vi "read_signal.vi"(8 "error in (no error)":errorcluster, 9 "Location":i32, 10 "Experiment Settings ID":i32, 11 "Dust Event ID":i32) -> (0 "error out":errorcluster, 3 "Signal Array":T1[](array[typedef]))   [LabVIEW 2012]
uses:
  Public API/Post_Signal.ctl
  Role ID.ctl
  Hardware ID.ctl
  <vilib>/addons/h5labview/H5F_mode.ctl
  <vilib>/addons/h5labview/polymorph/H5A_read_var.vi
  <vilib>/addons/h5labview/H5File.lvlib
  <vilib>/addons/h5labview/H5GroupObject.lvlib
  <vilib>/addons/h5labview/H5Attrib.lvlib
panel:
  out "size(s)":i32
  out "names":string[](array[string])
  # "Signal"
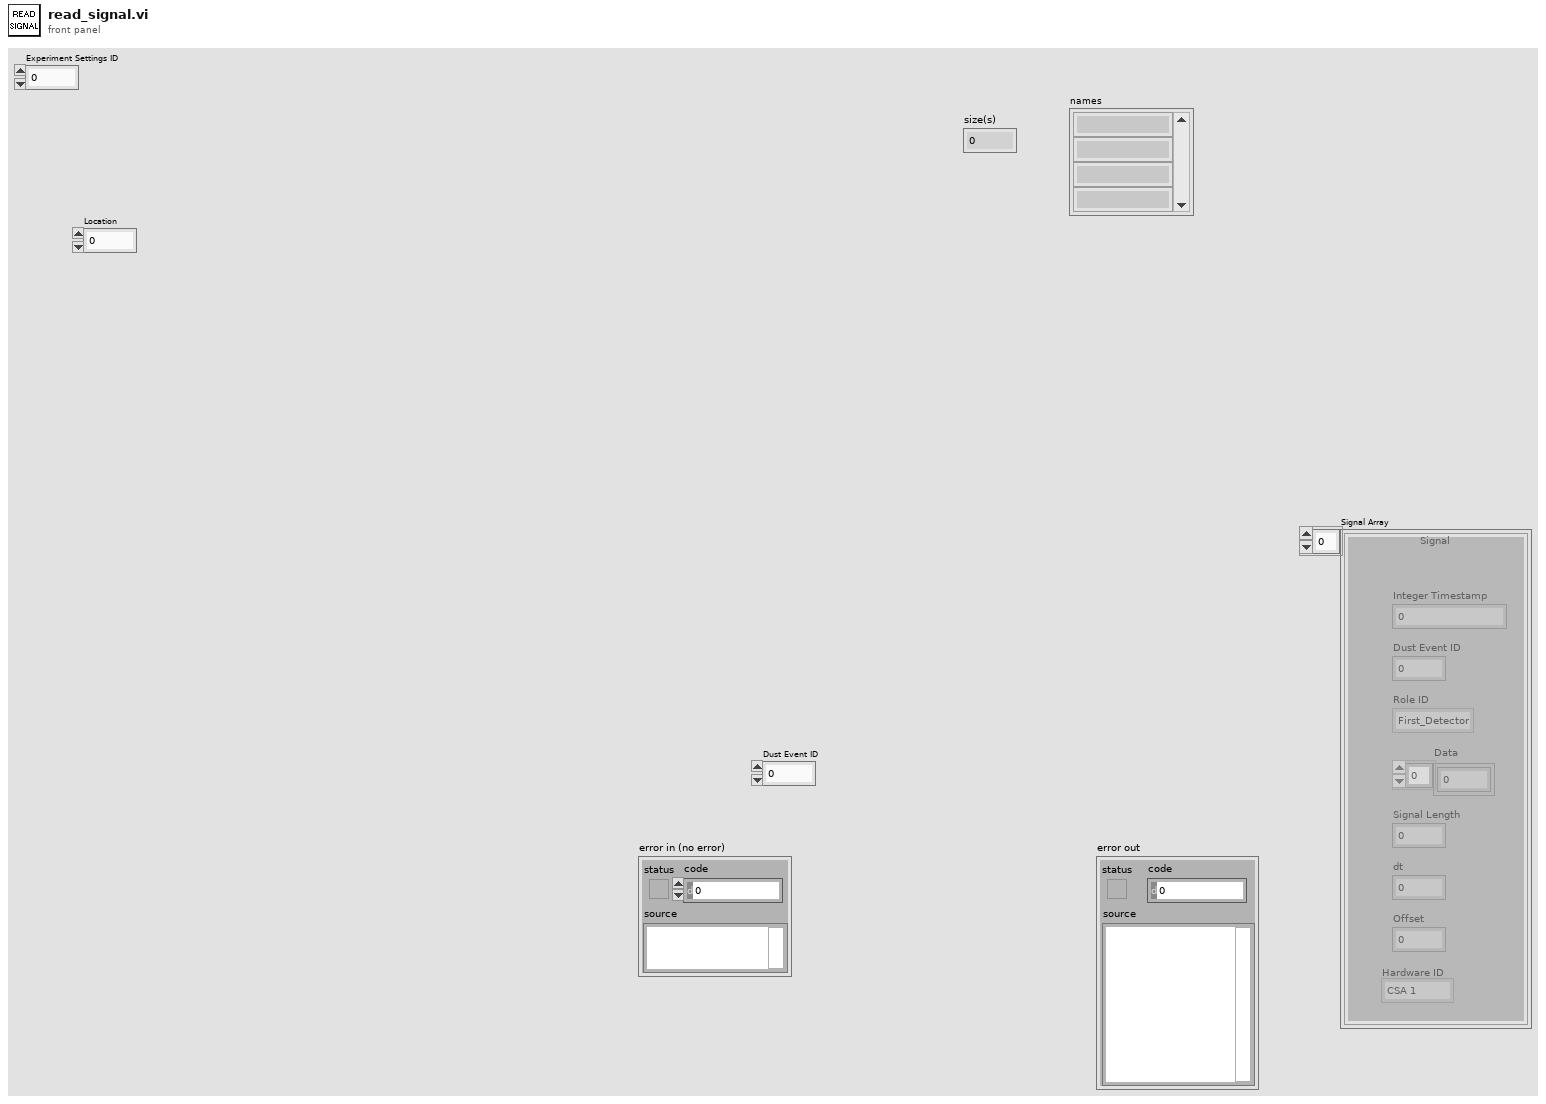
[diagram p1: front panel]
types:
  T1 = typedef "Post_Signal.ctl" = cluster{"Integer Timestamp":i64, "Dust Event ID":i64, "Role ID":T2, "Data":sgl[], "Signal Length":i32, "dt":sgl, "Offset":dbl, "Hardware ID":T3}
  T2 = typedef "Role ID.ctl" = enum16{"First_Detector", "Second_Detector", "Third_Detector", "LeCroy_CH1", "LeCroy_CH2", "LeCroy_CH3", "LeCroy_CH4", "PSU"}
  T3 = typedef "Hardware ID.ctl" = enum16{"Unknown", "CSA 1", "CSA 2", "CSA 3", "CSA 4", "CSA 5", "CSA 6"}
  T4 = typedef "H5File.lvlib/H5F_mode.ctl" = enum16{"read-only", "read-write", "overwrite", "create new", "open or create"}
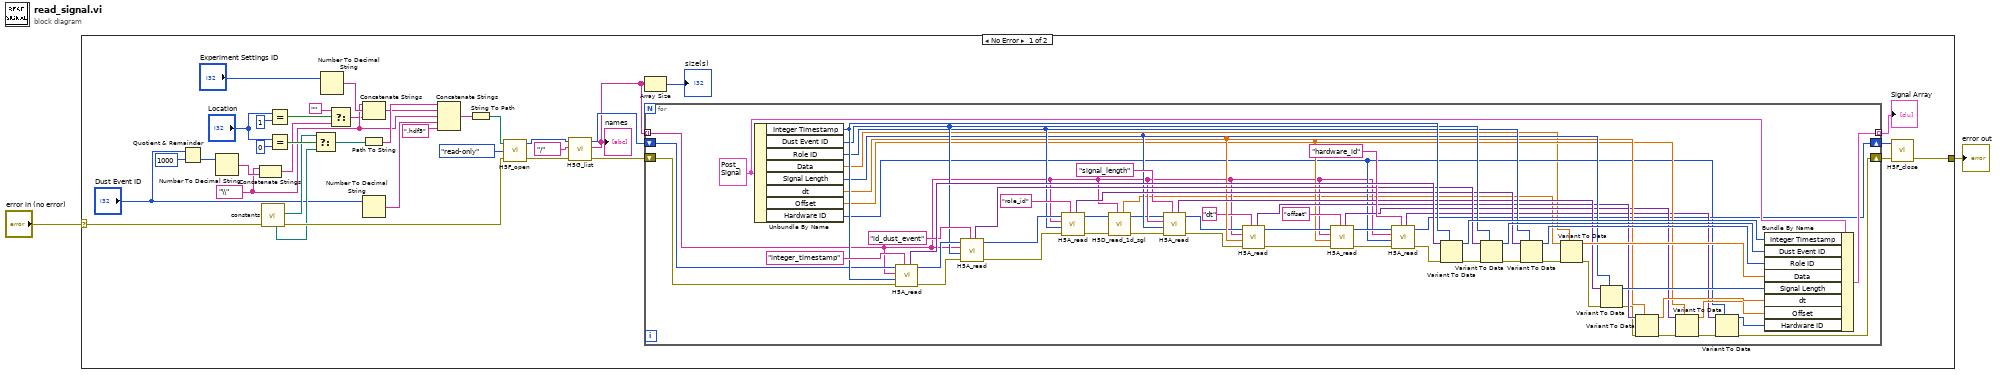
[diagram p0: block diagram]
diagram:
  n1 = case shown="No Error" "error in (no error)" {
    selector: "error in (no error)" -> [w35 w101]
    tunnel: [w40 w101] -> w2
    frame No Error {
      w6 = "\\"
      n2 = Quotient & Remainder(x="Dust Event ID", y=1000) -> (floor(x/y)=w11:i32)  [unwired: 1 out]
      n3 = Number To Decimal String(number=w11) -> (decimal integer string=w7:string)  [unwired: 1 in]
      n4 = Concatenate Strings(w6, w7) -> (w5:string)
      n5 = call "constants.vi"("error in (no error)"=w35) -> ("error out"=w36:errorcluster, "file path for Signal .hdf5 files"=w16:path, "file path for Processed Signal .hdf5 files"=w14:path)  [unwired: 4 in, 4 out]
      n6 = Equal?(x="Location", y=1) -> (x = y?=w8:bool)
      n7 = Equal?(x="Location", y=0 ("Location")) -> (x = y?=w17:bool)
      n8 = Select(t=w16, s=w17, f=w14) -> (s? t:f=w15:path)
      n9 = Number To Decimal String(number="Experiment Settings ID") -> (decimal integer string=w22:string)  [unwired: 1 in]
      n10 = Select(t="", s=w8, f=w5) -> (s? t:f=w3:string)
      n11 = Path To String(path=w15) -> (string=w21:string)
      n12 = Concatenate Strings(w6, w22, w3) -> (w20:string)
      n13 = Number To Decimal String(number="Dust Event ID") -> (decimal integer string=w37:string)  [unwired: 1 in]
      n14 = Concatenate Strings(w21, w20, w6, w37, ".hdf5") -> (w39:string)
      n15 = String To Path(string=w39) -> (path=w34:path)
      n16 = call <vilib>:"H5F_open.vi"("error in (no error)"=w36, "mode"=H5F_mode."read-only", "path"=w34) -> ("error out"=w31:errorcluster, "ref"=w32:i32)  [unwired: 1 in]
      n17 = call <vilib>:"H5G_list.vi"("error in (no error)"=w31, "group"="/", "ref"=w32) -> ("error out"=w29:errorcluster, "names"=w23:string[], "ref out"=w28:i32)  [unwired: 1 in, 1 out]
      "names" <- w23
      n18 = Array Size(array=w23) -> (size(s)=→"size(s)":i32)
      n19 = for {
        shift-right: [w48] -> w27
        shift-left: w29 -> [w91]
        shift-right: [w53] -> w26
        shift-left: w28 -> [w92]
        tunnel: [w98] -> w25 mode=indexing
        tunnel: w23 -> [w45] mode=indexing
        w100 = T1 {"Integer Timestamp"=0, "Dust Event ID"=0, "Role ID"=enum."First_Detector", "Data"=[], "Signal Length"=0, "dt"=0.0, "Offset"=0.0, "Hardware ID"=enum."CSA 1"} ("Post_Signal 2")
        n20 = Unbundle By Name(w100) -> ("Integer Timestamp"=w96:i64, "Dust Event ID"=w86:i64, "Role ID"=w79:T2, "Data"=w47:sgl[], "Signal Length"=w73:i32, "dt"=w69:sgl, "Offset"=w59:dbl, "Hardware ID"=w50:T3)
        n21 = call-poly <vilib>:"H5A_read.vi"("attrib_name"="integer_timestamp", "error in (no error)"=w91, "default"=w96, "obj_name"=w45, "ref"=w92) -> ("error out"=w88:errorcluster, "ref out"=w90:i32, "value"=w95:variant)  [unwired: 2 in]
        n22 = call-poly <vilib>:"H5A_read.vi"("attrib_name"="id_dust_event", "error in (no error)"=w88, "default"=w86, "obj_name"=w45, "ref"=w90) -> ("error out"=w83:errorcluster, "ref out"=w82:i32, "value"=w87:variant)  [unwired: 2 in]
        n23 = call-poly <vilib>:"H5A_read.vi"("attrib_name"="role_id", "error in (no error)"=w83, "default"=w79, "obj_name"=w45, "ref"=w82) -> ("error out"=w42:errorcluster, "ref out"=w46:i32, "value"=w80:variant)  [unwired: 2 in]
        n24 = call "H5D_read_1d_sgl.vi"("name"=w45, "error in (no error)"=w42, "ref"=w46) -> ("error out"=w41:errorcluster, "ref out"=w44:i32, "data"=w43:sgl[])  [unwired: 4 in]
        n25 = call-poly <vilib>:"H5A_read.vi"("attrib_name"="signal_length", "error in (no error)"=w41, "default"=w73, "obj_name"=w45, "ref"=w44) -> ("error out"=w65:errorcluster, "ref out"=w66:i32, "value"=w74:variant)  [unwired: 2 in]
        n26 = call-poly <vilib>:"H5A_read.vi"("attrib_name"="dt", "error in (no error)"=w65, "default"=w69, "obj_name"=w45, "ref"=w66) -> ("error out"=w62:errorcluster, "ref out"=w63:i32, "value"=w70:variant)  [unwired: 2 in]
        n27 = call-poly <vilib>:"H5A_read.vi"("attrib_name"="offset", "error in (no error)"=w62, "default"=w59, "obj_name"=w45, "ref"=w63) -> ("error out"=w55:errorcluster, "ref out"=w56:i32, "value"=w60:variant)  [unwired: 2 in]
        n28 = call-poly <vilib>:"H5A_read.vi"("attrib_name"="hardware_id", "error in (no error)"=w55, "default"=w50, "obj_name"=w45, "ref"=w56) -> ("error out"=w52:errorcluster, "ref out"=w53:i32, "value"=w54:variant)  [unwired: 2 in]
        n29 = Variant To Data(error in=w52, type=w96, Variant=w95) -> (data=w94:i64, error out=w84:errorcluster)
        n30 = Variant To Data(error in=w84, type=w86, Variant=w87) -> (data=w85:i64, error out=w77:errorcluster)
        n31 = Variant To Data(error in=w77, type=w79, Variant=w80) -> (data=w78:T2, error out=w76:errorcluster)
        n32 = Variant To Data(error in=w76, type=w47, Variant=w43) -> (data=w99:sgl[], error out=w72:errorcluster)
        n33 = Variant To Data(error in=w72, type=w73, Variant=w74) -> (data=w71:i32, error out=w67:errorcluster)
        n34 = Variant To Data(error in=w67, type=w69, Variant=w70) -> (data=w68:sgl, error out=w57:errorcluster)
        n35 = Variant To Data(error in=w57, type=w59, Variant=w60) -> (data=w58:dbl, error out=w51:errorcluster)
        n36 = Variant To Data(error in=w51, type=w50, Variant=w54) -> (data=w49:T3, error out=w48:errorcluster)
        n37 = Bundle By Name(cluster=w100, "Integer Timestamp"=w94, "Dust Event ID"=w85, "Role ID"=w78, "Data"=w99, "Signal Length"=w71, "dt"=w68, "Offset"=w58, "Hardware ID"=w49) -> (w98:T1)
      }
      "Signal Array" <- w25
      n38 = call <vilib>:"H5F_close.vi"("error in (no error)"=w27, "ref"=w26) -> ("error out"=w40:errorcluster)  [unwired: 3 in]
    }
    frame Error {
    }
  }
  "error out" <- w2
